vi "GetStatistics_Array.vi"(9 "n":i32[](array[numeric]), 10 "sum_X^2":dbl[][](array[numeric]), 11 "sum_X":dbl[][](array[numeric])) -> (3 "Table":dbl[][](array[numeric]))   [LabVIEW 2012]
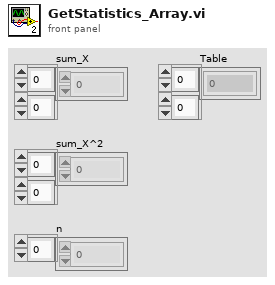
[diagram p1: front panel]
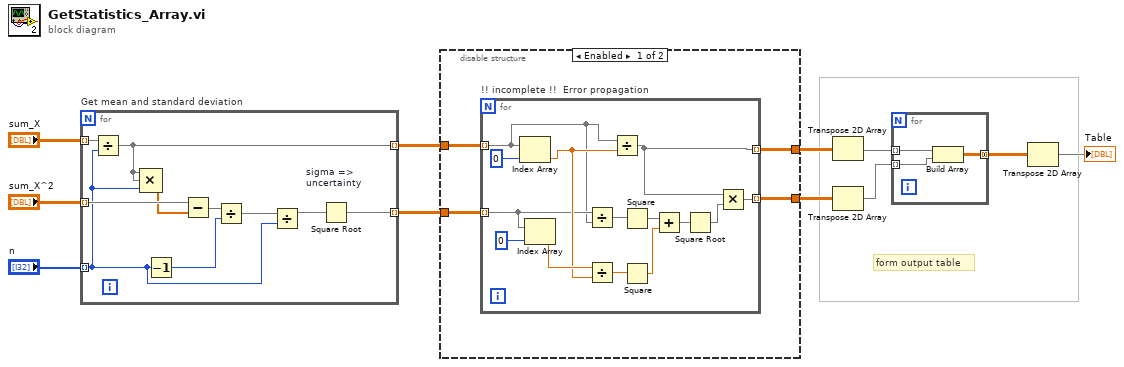
[diagram p0: block diagram]
diagram:
  # "form output table"
  n1 = for "Get mean and standard deviation" {
    tunnel: "sum_X" -> [w16] mode=indexing
    tunnel: [w14] -> w4 mode=indexing
    tunnel: "sum_X^2" -> [w21] mode=indexing
    tunnel: "n" -> [w12] mode=indexing
    tunnel: [w17] -> w5 mode=indexing
    n2 = Divide(x=w16, y=w12) -> (x/y=w14:dbl[])
    n3 = Compound Arithmetic op=MULTIPLY(w14, w14, w12) -> (w15:dbl[])
    n4 = Decrement(x=w12) -> (x-1=w20:i32)
    n5 = Subtract(x=w21, y=w15) -> (x-y=w18:dbl[])
    n6 = Divide(x=w18, y=w20) -> (x/y=w19:dbl[])
    n7 = Divide "sigma => \nuncertainty"(x=w19, y=w12) -> (x/y=w13:dbl[])
    n8 = Square Root(x=w13) -> (sqrt(x)=w17:dbl[])
  }
  n9 = disable-structure shown="Enabled" {
    disable-tunnel: [w25 w40] -> w6
    disable-tunnel: w4 -> [w24 w40]
    disable-tunnel: w5 -> [w23 _]
    disable-tunnel: [w22 _] -> w7
    frame Enabled {
      n10 = for "!! incomplete !!  Error propagation" {
        tunnel: w24 -> [w32] mode=indexing
        tunnel: [w26] -> w25 mode=indexing
        tunnel: w23 -> [w33] mode=indexing
        tunnel: [w27] -> w22 mode=indexing
        n11 = Index Array(array=w32, index=0) -> (element=w36:dbl)
        n12 = Index Array(array=w33, index=0) -> (element=w37:dbl)
        n13 = Divide(x=w33, y=w32) -> (x/y=w34:dbl[])
        n14 = Divide(x=w37, y=w36) -> (x/y=w35:dbl)
        n15 = Divide(x=w32, y=w36) -> (x/y=w26:dbl[])
        n16 = Square(x=w34) -> (x^2=w31:dbl[])
        n17 = Square(x=w35) -> (x^2=w30:dbl)
        n18 = Add(x=w31, y=w30) -> (x+y=w29:dbl[])
        n19 = Square Root(x=w29) -> (sqrt(x)=w28:dbl[])
        n20 = Multiply(x=w26, y=w28) -> (x*y=w27:dbl[])
      }
    }
    frame Disabled {
    }
  }
  n21 = Transpose 2D Array(2D array=w6) -> (transposed array=w8:dbl[][])
  n22 = Transpose 2D Array(2D array=w7) -> (transposed array=w9:dbl[][])
  n23 = for {
    tunnel: w8 -> [w43] mode=indexing
    tunnel: w9 -> [w42] mode=indexing
    tunnel: [w41] -> w10 mode=concatenating
    n24 = Build Array(w43, w42) -> (w41:dbl[][])
  }
  n25 = Transpose 2D Array(2D array=w10) -> (transposed array=→"Table":dbl[][])
